vi "GetEndDate.vi"(8 "error in":errorcluster, 11 "SequenceRun in":refnum<class "SequenceRun.lvclass">) -> (0 "error out":errorcluster, 2 "EndDate":timestamp, 3 "SequenceRun out":refnum<class "SequenceRun.lvclass">)   [LabVIEW 2021, in "ProligentXMLGenerator.lvlib" / "SequenceRun.lvclass"]
doc: "Defines the actual date where the sequence run ended.\nIf 'SequenceExecutionStatus' is equal to 'NOT_COMPLETED' this value must be ommited.\nSequenceRunId must have been provided to allow sequence run updates through DIT increment.\nThis value must be greater or equal than StartDate.\n\nNote that the if the Data Warehouse already contains this sequence run but it is not already\nclosed, the EndDate written in the Data Warehouse will be set according to the following rule: EndDate(in database) = StartDate(in database) + (EndDate(from xml) - StartDate(from xml)).\n\nThis value is restricted to \"1900-01-01T00:00:00Z\" -\"2100-01-01T00:00:00Z\"."
uses:
  SequenceRun.lvclass
  SequenceRun.lvclass/SequenceRun.ctl
  Base/DateTime/DateTime.lvclass
  Base/Attribute/Attribute.lvclass
  C:/Projects/proligent-xml-generator-labview/src/ProligentXMLGenerator/Base/Attribute/Attribute.lvclass
  C:/Projects/proligent-xml-generator-labview/src/ProligentXMLGenerator/Base/DateTime/DateTime.lvclass
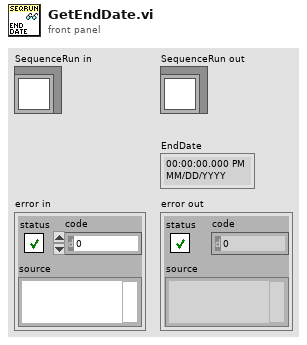
[diagram p1: front panel]
types:
  T1 = typedef "ProligentXMLGenerator.lvlib/SequenceRun.lvclass/Data.ctl" = cluster{"Name":string, "StepRuns":refnum<class "StepRun.lvclass">[], "Characteristics":refnum<class "Characteristic.lvclass">[], "Documents":refnum<class "Document.lvclass">[], "FailureReferences":refnum<class "FailureReference.lvclass">[], "CustomData":refnum<class "CustomData.lvclass">, "StartDate":refnum<class "DateTime.lvclass">, "EndDate":refnum<class "DateTime.lvclass">, "SequenceExecutionStatus":refnum<class "ExecutionStatus.lvclass">, "SequenceRunId":refnum<class "Guid.lvclass">, "SequenceFullName":refnum<class "SequenceFullName.lvclass">, "SequenceVersion":refnum<class "NonEmptyString_64.lvclass">, "StationFullName":refnum<class "FullName.lvclass">, "User":refnum<class "NonEmptyString_255.lvclass">, "TimeZoneInfoId":string}
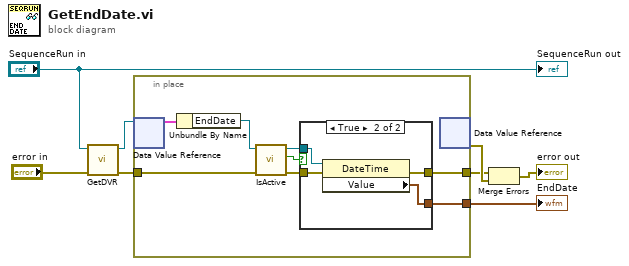
[diagram p0: block diagram]
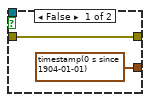
[diagram p2: hidden frame]
diagram:
  n1 = call "GetDVR.vi"("error in"="error in", "SequenceRun"="SequenceRun in") -> ("error out"=w2:errorcluster, "DVRReference"=w7:refnum<data-value>)  [unwired: 8 in]
  n2 = in-place "In Place Element Structure" {
    in-place-border: [w15] -> w6
    in-place-border: w2 -> [w11]
    in-place-border: [w14] -> w1
    n3 = in-place-dvr #1(w7) -> (w16:T1)  [unwired: 1 out]
    n4 = Unbundle By Name(w16) -> ("EndDate"=w13:refnum<class "DateTime.lvclass">)
    n5 = call "IsActive.vi"("error in"=w11, "Attribute in"=w13) -> ("error out"=w10:errorcluster, "IsActive"=w9:bool, "Attribute in"=w12:refnum<class "DateTime.lvclass">)  [unwired: 7 in]
    n6 = case shown="True" w9 {
      tunnel: [timestamp(0 s since 1904-01-01) ("Value") w22] -> w15
      tunnel: [w17 w21] -> w14
      tunnel: w12 -> [_ w20]
      tunnel: w10 -> [w17 w19]
      frame False {
      }
      frame True {
        n7 = property on="Property Node" class="DateTime"(reference=w20, error in=w19) -> (error out=w21:errorcluster, "Value"=w22:timestamp)  [unwired: 1 out]
      }
    }
    n8 = in-place-dvr #1() -> (w8:errorcluster)  [unwired: 1 in, 1 out]
  }
  "EndDate" <- w6
  n9 = Merge Errors(w1, w8) -> (→"error out":errorcluster)
  "SequenceRun out" <- "SequenceRun in"
